vi "tracking2.vi"(4 "x 2":dbl=10.0, 6 "lane keep":bool, 7 "str_gain":dbl=0.9 format="%#_13g", 8 "Numeric 2":dbl=10.0 format="%#_13g", 9 "reset path":bool, 11 "xt":dbl) -> (3 "handle":dbl=-3.32529799262397)   [LabVIEW 2015]
uses:
  G_SEN.vi
  G_ALL.vi
  G_LCM.vi
panel:
  out "lanedist":dbl
  out "idxx":dbl[](array[numeric])
  out "idx":dbl
  in  "y 2":dbl=42.0
  out "XY Graph 2":cluster{"Y":dbl[], "Y":dbl[]}[](graph)=[{"Y"=array[11233 elements], "Y"=array[11233 elements]}, {"Y"=[-0.0, 0.0027755521495791413, 0.011103235155417224, 0.024986130588096955, 0.04442938073793812, 0.0694401981527264, 0.10002787904836907, 0.13620382065079895, 0.17798154254490584, 0.22537671212434418, 0.2784071742547809, 0.3370929852830926, 0.40145645154536425, 0.4715221725490224, 0.5473170890276435, 0.6288705360921867, 0.7162143017295008, 0.8093826909282242, 0.9084125957438758, 1.0133435716494645, 1.1242179205557647, 1.2410807809266515, 1.3639802254602955, 1.4929673668571652, 1.6280964722509026, 1.769425086939485, 1.9170141681219874, 2.0709282294217246, 2.2312354970611636, 2.3980080786478197, 2.5713221456362234], "Y"=[0.0, 0.5, 1.0, 1.5, 2.0, 2.5, 3.0, 3.5, 4.0, 4.5, 5.0, 5.5, 6.0, 6.5, 7.0, 7.5, 8.0, 8.5, 9.0, 9.5, 10.0, 10.5, 11.0, 11.5, 12.0, 12.5, 13.0, 13.5, 14.0, 14.5, 15.0]}, {"Y"=[-0.40885366553013214], "Y"=[0.1442103688222703]}, {"Y"=array[212 elements], "Y"=array[212 elements]}, {"Y"=[-0.925, -0.925, -0.925, -0.6775, -0.6775, -0.925, -0.925, -0.925, -0.925, -0.6775, -0.6775, -0.925, -0.925, -0.925, 0.9025, 0.9025, 0.9025, 0.6775, 0.6775, 0.9025, 0.9025, 0.9025, 0.9025, 0.6775, 0.6775, 0.9025, 0.9025, 0.9025, -0.925], "Y"=[-0.75, -0.224, 0.224, 0.224, -0.224, -0.224, 0.224, 2.415, 2.885, 2.885, 2.415, 2.415, 2.885, 3.5, 3.5, 2.885, 2.415, 2.415, 2.885, 2.885, 2.415, 0.224, -0.224, -0.224, 0.224, 0.224, -0.224, -0.75, -0.75]}, {"Y"=[0.0, 0.0, 0.0, 0.0, 0.0, 0.0, 0.0, 0.0, 0.0, 0.0], "Y"=[0.0, 0.5, 1.0, 1.5, 2.0, 2.5, 3.0, 3.5, 4.0, 4.5]}, {"Y"=[1.41796875, 1.3798326583616436, 1.3415997434556484, 1.3032752327956258, 1.2648643538951874, 1.226372334267944, 1.1878044014275073, 1.1491657828874886, 1.110461706161499, 1.07169739876315], "Y"=[0.0, 0.5, 1.0, 1.5, 2.0, 2.5, 3.0, 3.5, 4.0, 4.5]}, {"Y"=[-2.5234375, -2.5105986626297234, -2.4915998479127883, -2.466420726940036, -2.4350409708023073, -2.3974402505904435, -2.3535982373952864, -2.303494602307677, -2.247109016418457, -2.184421150818467], "Y"=[0.0, 0.5, 1.0, 1.5, 2.0, 2.5, 3.0, 3.5, 4.0, 4.5]}, {"Y"=[0.0, 0.0, 0.0, 0.0, 0.0, 0.0, 0.0, 0.0, 0.0, 0.0, 0.0, 0.0, 0.0, 0.0, 0.0, 0.0, 0.0, 0.0, 0.0, 0.0], "Y"=[0.0, 0.5, 1.0, 1.5, 2.0, 2.5, 3.0, 3.5, 4.0, 4.5, 5.0, 5.5, 6.0, 6.5, 7.0, 7.5, 8.0, 8.5, 9.0, 9.5]}]
  out "dist":dbl[](array[numeric])
  out "y origin":dbl[](array[numeric])
  out "x origin":dbl[](array[numeric])
  out "heading":dbl[](array[numeric])
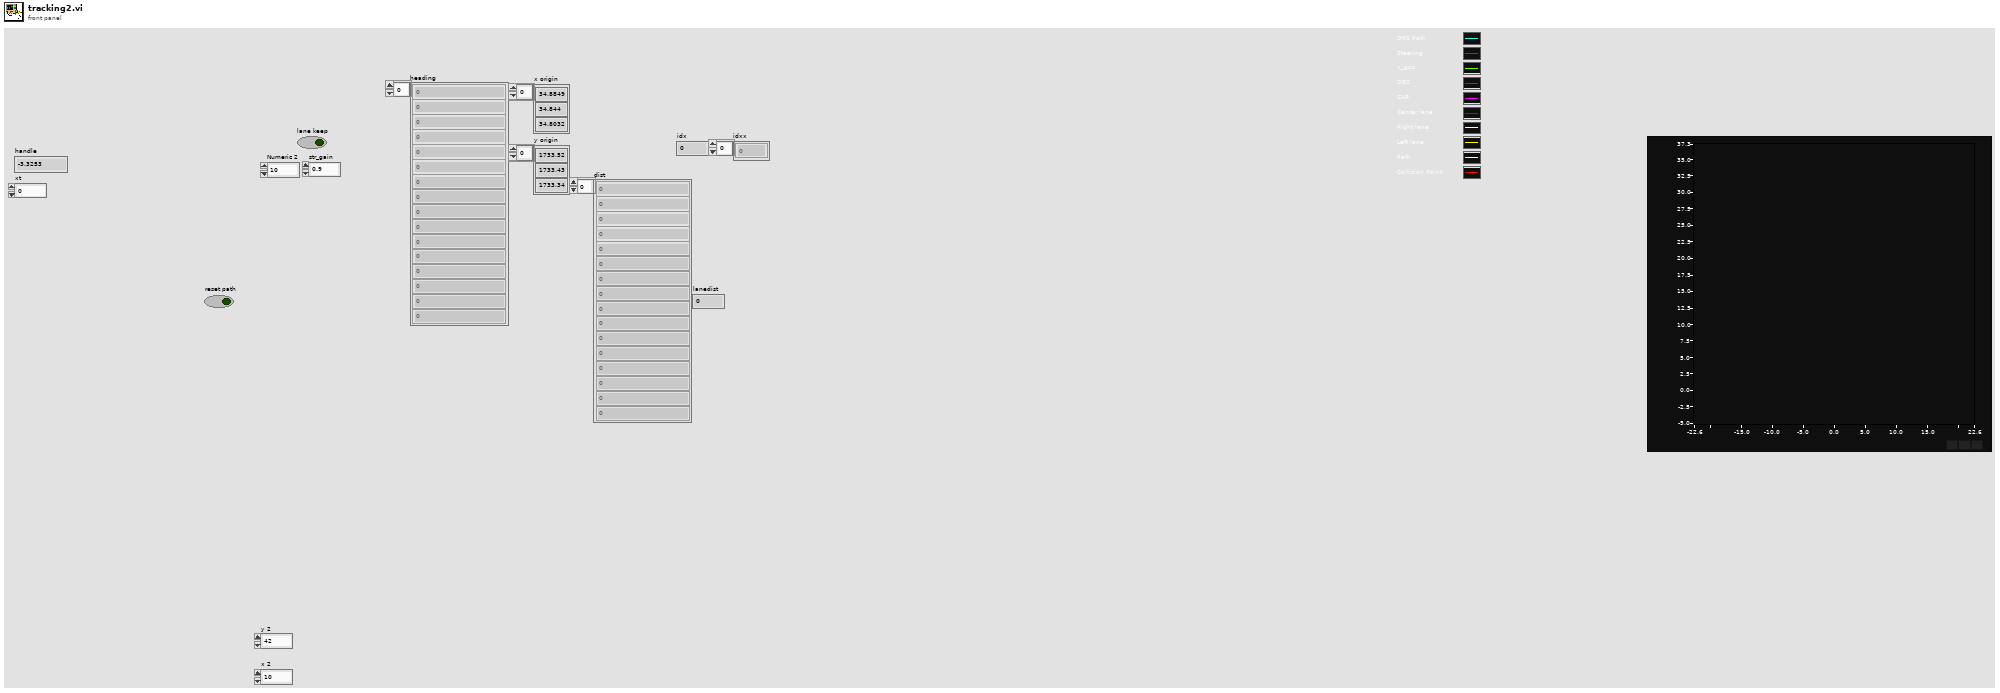
[diagram p1: front panel]
types:
  T1 = cluster{"Steer_input":dbl, "Steer_output":dbl, "VS_des":dbl, "VS_can":dbl, "heading":dbl, "auto":bool, "run":bool, "x":dbl, "y":dbl}
  T2 = cluster{"beep":bool, "duration (msec)":u32, "frequency (Hz)":u32}
  T3 = cluster{"C_Wheel base":dbl, "ratio_steer":dbl, "Overall width":dbl, "af":dbl, "turn radius":dbl, "eval":dbl, "ap":dbl, "an":dbl, "Vmax":dbl, "mu":dbl, "Vlast":dbl}
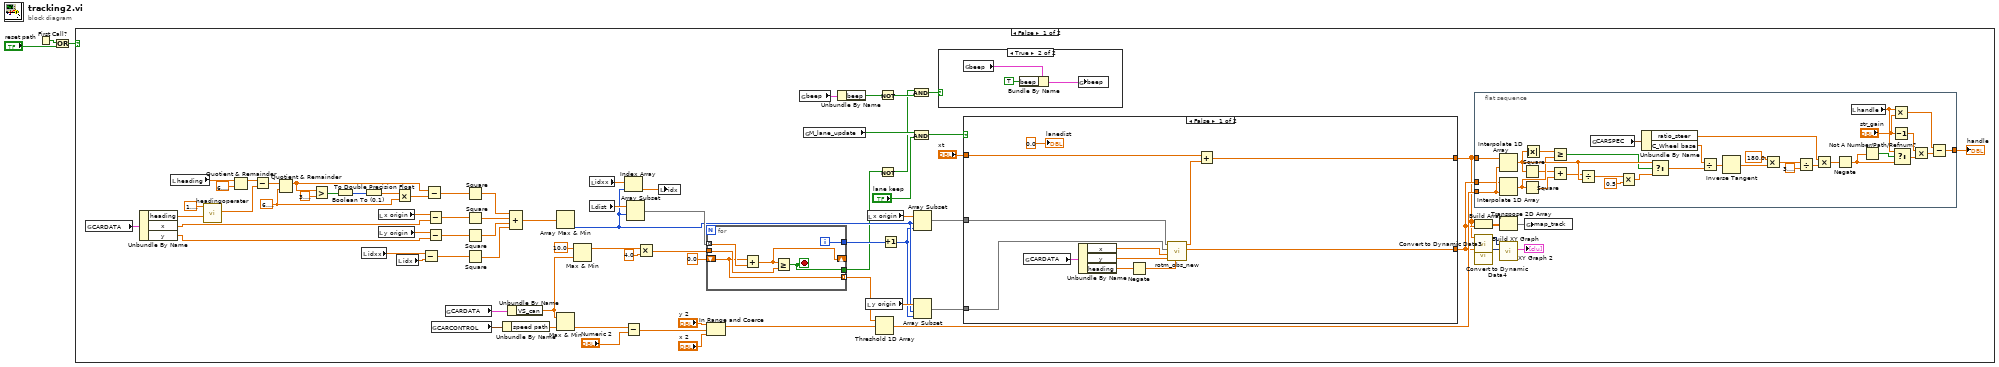
[diagram p0: block diagram]
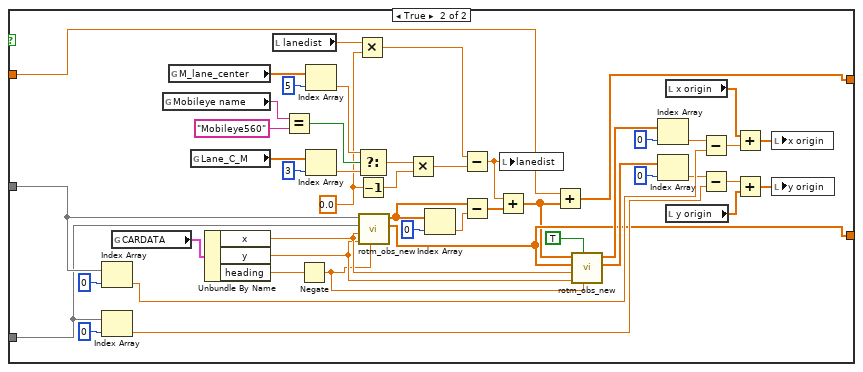
[diagram p3: hidden frame]
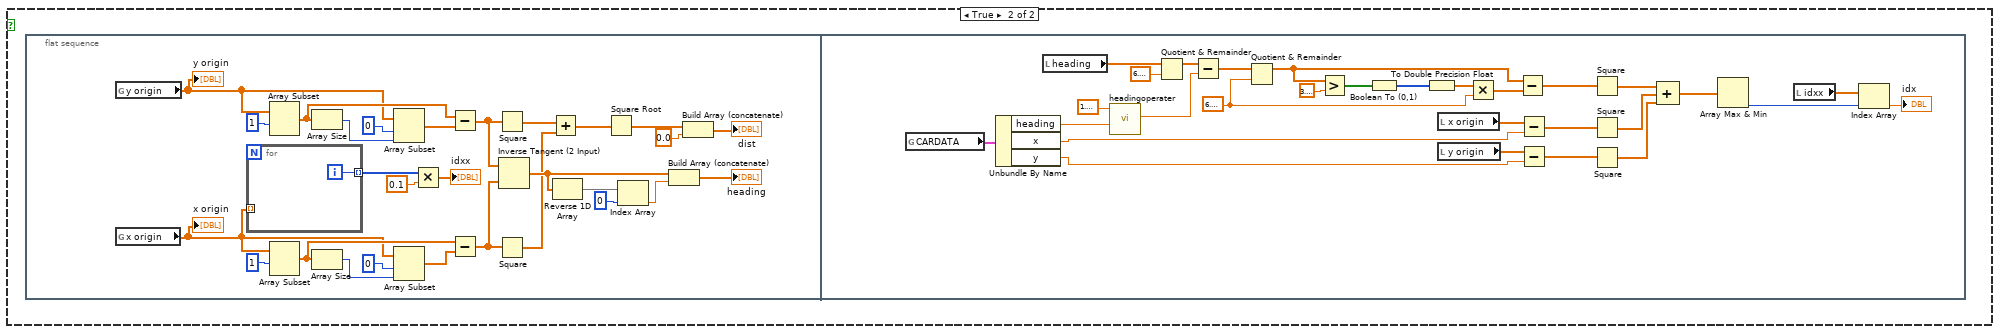
[diagram p4: hidden frame]
diagram:
  n1 = First Call?() -> (First Call?: T/F=w3:bool)
  n2 = Or(x=w3, y="reset path") -> (x .or. y?=w2:bool)
  n3 = case shown="False" w2 {
    frame False {
      w64 = 6.283185307179586
      n4 = global read "G_ALL.vi" "CARDATA"() -> (w11:T1)
      n5 = Unbundle By Name(w11) -> ("heading"=w58:dbl, "x"=w79:dbl, "y"=w77:dbl)
      n6 = local read "heading"() -> (w69:dbl[])
      n7 = call "headingoperater.vi"("h1"=w58, "h2"=1.5707963267948966) -> ("h2-h1"=w55:dbl)  [unwired: 8 in, 1 out]
      n8 = Quotient & Remainder(x=w69, y=6.283185307179586) -> (x-y*floor(x/y)=w70:dbl[])  [unwired: 1 out]
      n9 = Subtract(x=w70, y=w55) -> (x-y=w71:dbl[])
      n10 = Quotient & Remainder(x=w71, y=w64) -> (x-y*floor(x/y)=w72:dbl[])  [unwired: 1 out]
      n11 = Greater?(x=w72, y=3.141592653589793) -> (0:w68:bool[])
      n12 = Boolean To (0,1)(Boolean=w68) -> (0, 1=w67:i16[])
      n13 = local read "idxx"() -> (w25:dbl[])
      n14 = To Double Precision Float(number=w67) -> (double precision float=w65:dbl[])
      n15 = local read "x origin"() -> (w78:dbl[])
      n16 = local read "y origin"() -> (w76:dbl[])
      n17 = Multiply(x=w65, y=w64) -> (x*y=w66:dbl[])
      n18 = local read "idx"() -> (w26:dbl)
      n19 = Subtract(x=w25, y=w26) -> (x-y=w24:dbl[])
      n20 = Subtract(x=w72, y=w66) -> (x-y=w63:dbl[])
      n21 = Subtract(x=w78, y=w79) -> (x-y=w61:dbl[])
      n22 = Subtract(x=w76, y=w77) -> (x-y=w62:dbl[])
      n23 = global read "G_ALL.vi" "CARCONTROL"() -> (w5:cluster{"speed path":dbl, "speed limit":dbl})
      n24 = global read "G_ALL.vi" "CARDATA"() -> (w10:T1)
      n25 = Square(x=w63) -> (x^2=w60:dbl[])
      n26 = Square(x=w61) -> (x^2=w57:dbl[])
      n27 = Square(x=w62) -> (x^2=w56:dbl[])
      n28 = Square(x=w24) -> (x^2=w23:dbl[])
      n29 = Unbundle By Name(w5) -> ("speed path"=w4:dbl)
      n30 = Unbundle By Name(w10) -> ("VS_can"=w9:dbl)
      n31 = Compound Arithmetic op=ADD(w60, w57, w56, w23) -> (w59:dbl[])
      n32 = Array Max & Min(array=w59) -> (min index (indices)=w21:i32)  [unwired: 3 out]
      n33 = Max & Min(x=w9, y=w4) -> (min(x,y)=w29:dbl)  [unwired: 1 out]
      n34 = Max & Min(x=10.0, y=w9) -> (max(x,y)=w52:dbl)  [unwired: 1 out]
      n35 = local read "idxx"() -> (w22:dbl[])
      n36 = local read "dist"() -> (w54:dbl[])
      n37 = Index Array(array=w22, index=w21) -> (element=w20:dbl)
      n38 = Subtract(x=w29, y="Numeric 2") -> (x-y=w28:dbl)
      n39 = Array Subset(array=w54, index=w21) -> (w50:dbl[])  [unwired: 1 in]
      n40 = Multiply(x=w52, y=4.0) -> (x*y=w49:dbl)
      n41 = local write "idx"(w20) -> ()
      n42 = for {
        tunnel: w50 -> [w181] mode=indexing
        tunnel: w49 -> [w179]
        shift-right: [w180] -> _
        shift-left: 0.0 -> [w177]
        tunnel: [w178] -> w47
        tunnel: [w177] -> w31 mode=indexing
        tunnel: [w176] -> w13
        i -> [w178]
        stop <- w176 stop-if-true
        n43 = Add(x=w177, y=w181) -> (x+y=w180:dbl)
        n44 = Greater Or Equal?(x=w180, y=w179) -> (x >= y?=w176:bool)
      }
      n45 = In Range and Coerce(upper limit="y 2", x=w28, lower limit="x 2") -> (coerced(x)=w36:dbl)  [unwired: 1 out]
      n46 = global read "G_ALL.vi" "beep"() -> (w7:T2)
      n47 = global read "G_SEN.vi" "M_lane_update"() -> (w42:bool)
      n48 = Unbundle By Name(w7) -> ("beep"=w6:bool)
      n49 = local read "y origin"() -> (w43:dbl[])
      n50 = local read "x origin"() -> (w44:dbl[])
      n51 = Threshold 1D Array(2:w36, 3:w31) -> (0:w37:dbl)  [unwired: 1 in]
      n52 = Not(x=w6) -> (.not. x?=w17:bool)
      n53 = Not(x=w13) -> (.not. x?=w12:bool)
      n54 = Increment(x=w47) -> (x+1=w14:i32)
      n55 = And(x=w12, y=w17) -> (x .and. y?=w16:bool)
      n56 = And(x=w42, y="lane keep") -> (x .and. y?=w41:bool)
      n57 = Array Subset(array=w44, index=w21, length=w14) -> (w46:dbl[])
      n58 = Array Subset(array=w43, index=w21, length=w14) -> (w15:dbl[])
      n59 = case shown="True" w16 {
        frame False {
        }
        frame True {
          n60 = global read "G_ALL.vi" "beep"() -> (w82:T2)
          n61 = Bundle By Name(cluster=w82, "beep"=TRUE) -> (w81:T2)
          n62 = global write "G_ALL.vi" "beep"(w81) -> ()
        }
      }
      n63 = case shown="False" w41 {
        tunnel: w46 -> [w123 w154]
        tunnel: w15 -> [w122 w152]
        tunnel: [w120 w137] -> w32
        tunnel: [w121 w139] -> w33
        tunnel: "xt" -> [w118 w136]
        frame False {
          n64 = global read "G_ALL.vi" "CARDATA"() -> (w116:T1)
          n65 = Unbundle By Name(w116) -> ("x"=w126:dbl, "y"=w125:dbl, "heading"=w127:dbl)
          n66 = Negate(x=w127) -> (-x=w124:dbl)
          n67 = call "rotm_obs_new.vi"("angle[rad]"=w124, "y0"=w125, "x0"=w126, "y"=w122, "x"=w123) -> ("rot*(y-y0) 2"=w121:dbl[], "rot*(x-x0)"=w119:dbl[])  [unwired: 3 in, 2 out]
          n68 = Add(x=w118, y=w119) -> (x+y=w120:dbl[])
          "lanedist" <- 0.0
        }
        frame True {
          w134 = 0.0 ("x")
          n69 = Index Array(array=w154, index=0) -> (element=w150:dbl)
          n70 = Index Array(array=w152, index=0) -> (element=w146:dbl)
          n71 = global read "G_ALL.vi" "CARDATA"() -> (w128:T1)
          n72 = global read "G_LCM.vi" "Mobileye name"() -> (w167:string)
          n73 = global read "G_SEN.vi" "M_lane_center"() -> (w162:dbl[])
          n74 = global read "G_SEN.vi" "Lane_C_M"() -> (w169:dbl[])
          n75 = Unbundle By Name(w128) -> ("x"=w160:dbl, "y"=w159:dbl, "heading"=w175:dbl)
          n76 = local read "lanedist"() -> (w135:dbl)
          n77 = Equal?(x=w167, y="Mobileye560") -> (x = y?=w165:bool)
          n78 = Negate(x=w175) -> (-x=w158:dbl)
          n79 = Index Array(array=w162, index=5) -> (element=w161:dbl)
          n80 = Index Array(array=w169, index=3) -> (element=w164:dbl)
          n81 = Multiply(x=w135, y=w134) -> (x*y=w131:dbl)
          n82 = Select(t=w161, s=w165, f=w164) -> (s? t:f=w133:dbl)
          n83 = Decrement(x=w134) -> (x-1=w132:dbl)
          n84 = call "rotm_obs_new.vi"("angle[rad]"=w158, "y0"=w159, "x0"=w160, "y"=w152, "x"=w154) -> ("rot*(y-y0) 2"=w139:dbl[], "rot*(x-x0)"=w172:dbl[])  [unwired: 3 in, 2 out]
          n85 = Multiply(x=w133, y=w132) -> (x*y=w130:dbl)
          n86 = Index Array(array=w172, index=0) -> (element=w173:dbl)
          n87 = Subtract(x=w131, y=w130) -> (x-y=w129:dbl)
          n88 = Subtract(x=w172, y=w173) -> (x-y=w171:dbl[])
          n89 = Add(x=w129, y=w171) -> (x+y=w138:dbl[])
          n90 = local write "lanedist"(w129) -> ()
          n91 = Add(x=w136, y=w138) -> (x+y=w137:dbl[])
          n92 = call "rotm_obs_new.vi"("angle[rad]"=w158, "reverse"=TRUE, "y0"=w159, "x0"=w160, "y"=w139, "x"=w138) -> ("rot*(y-y0) 2"=w148:dbl[], "rot*(x-x0)"=w157:dbl[])  [unwired: 2 in, 2 out]
          n93 = Index Array(array=w157, index=0) -> (element=w151:dbl)
          n94 = Index Array(array=w148, index=0) -> (element=w147:dbl)
          n95 = local read "x origin"() -> (w144:dbl[])
          n96 = local read "y origin"() -> (w142:dbl[])
          n97 = Subtract(x=w151, y=w150) -> (x-y=w145:dbl)
          n98 = Subtract(x=w147, y=w146) -> (x-y=w143:dbl)
          n99 = Add(x=w144, y=w145) -> (x+y=w141:dbl[])
          n100 = Add(x=w143, y=w142) -> (x+y=w140:dbl[])
          n101 = local write "x origin"(w141) -> ()
          n102 = local write "y origin"(w140) -> ()
        }
      }
      n103 = flat-sequence {
        tunnel: w37 -> [w113]
        tunnel: w33 -> [w112]
        tunnel: w32 -> [w93]
        tunnel: [w86] -> w30
        frame #0 {
          n104 = Interpolate 1D Array(1:w113, 2:w93) -> (0:w115:dbl)
          n105 = Interpolate 1D Array(1:w113, 2:w112) -> (0:w114:dbl)
          n106 = Square(x=w115) -> (x^2=w98:dbl)
          n107 = Square(x=w114) -> (x^2=w99:dbl)
          n108 = Absolute Value(x=w115) -> (abs(x)=w97:dbl)
          n109 = Greater Or Equal?(x=w97, y=w114) -> (x >= y?=w96:bool)
          n110 = Add(x=w98, y=w99) -> (x+y=w100:dbl)
          n111 = Divide(x=w100, y=w115) -> (x/y=w101:dbl)
          n112 = global read "G_ALL.vi" "CARSPEC"() -> (w85:T3)
          n113 = Multiply(x=w101, y=0.5) -> (x*y=w103:dbl)
          n114 = Unbundle By Name(w85) -> ("ratio_steer"=w84:dbl, "C_Wheel base"=w83:dbl)
          n115 = Select(t=w115, s=w96, f=w103) -> (s? t:f=w104:dbl)
          n116 = Divide(x=w83, y=w104) -> (x/y=w105:dbl)
          n117 = Inverse Tangent(1:w105) -> (0:w107:dbl)
          n118 = Multiply(x=180.0 ("y"), y=w107) -> (x*y=w108:dbl)
          n119 = Divide(x=w108, y=3.141592653589793) -> (x/y=w110:dbl)
          n120 = Multiply(x=w84, y=w110) -> (x*y=w111:dbl)
          n121 = Negate(x=w111) -> (-x=w94:dbl)
          n122 = local read "handle"() -> (w92:dbl)
          n123 = Not A Number/Path/Refnum?(number/path/refnum=w94) -> (NaN/Path/Refnum?=w95:bool)
          n124 = Multiply(x=w92, y="str_gain") -> (x*y=w88:dbl)
          n125 = Decrement(x="str_gain") -> (x-1=w90:dbl)
          n126 = Select(t=w92, s=w95, f=w94) -> (s? t:f=w89:dbl)
          n127 = Multiply(x=w90, y=w89) -> (x*y=w87:dbl)
          n128 = Subtract(x=w88, y=w87) -> (x-y=w86:dbl)
        }
      }
      n129 = Build Array(w32, w33) -> (w38:dbl[][])
      n130 = call "Convert to Dynamic Data3"("Array"=w32) -> ("Dynamic Data Type"=w40:dynamicdata)  [unwired: 3 in]
      n131 = call "Convert to Dynamic Data4"("Array"=w33) -> ("Dynamic Data Type"=w39:dynamicdata)  [unwired: 3 in]
      n132 = Transpose 2D Array(2D array=w38) -> (transposed array=w8:dbl[][])
      n133 = call "Build XY Graph"("Y Input"=w39, "X Input"=w40) -> ("XY Graph"=→"XY Graph 2":cluster{"X":dbl[], "Y":dbl[]}[])  [unwired: 8 in, 1 out]
      n134 = global write "G_ALL.vi" "map_track"(w8) -> ()
      "handle" <- w30
    }
    frame True {
      n135 = flat-sequence {
        frame #0 {
          n136 = global read "G_ALL.vi" "y origin"() -> (w182:dbl[])
          "y origin" <- w182
          n137 = global read "G_ALL.vi" "x origin"() -> (w183:dbl[])
          "x origin" <- w183
          n138 = for {
            tunnel: w183 -> [_] mode=indexing
            tunnel: [w210] -> w186 mode=indexing
            i -> [w210]
          }
          n139 = Array Subset(array=w182, index=1) -> (w204:dbl[])  [unwired: 1 in]
          n140 = Array Subset(array=w183, index=1) -> (w205:dbl[])  [unwired: 1 in]
          n141 = Array Size(array=w204) -> (size(s)=w201:i32)
          n142 = Array Size(array=w205) -> (size(s)=w208:i32)
          n143 = Array Subset(array=w182, index=0, length=w201) -> (w203:dbl[])
          n144 = Array Subset(array=w183, index=0, length=w208) -> (w206:dbl[])
          n145 = Multiply(x=w186, y=0.1) -> (x*y=→"idxx":dbl[])
          n146 = Subtract(x=w204, y=w203) -> (x-y=w194:dbl[])
          n147 = Subtract(x=w205, y=w206) -> (x-y=w193:dbl[])
          n148 = Square(x=w194) -> (x^2=w192:dbl[])
          n149 = Square(x=w193) -> (x^2=w191:dbl[])
          n150 = Inverse Tangent (2 Input)(1:w193, 2:w194) -> (0:w195:dbl[])
          n151 = Add(x=w192, y=w191) -> (x+y=w190:dbl[])
          n152 = Reverse 1D Array(array=w195) -> (reversed array=w199:dbl[])
          n153 = Square Root(x=w190) -> (sqrt(x)=w189:dbl[])
          n154 = Index Array(array=w199, index=0) -> (element=w197:dbl)
          n155 = Build Array (concatenate)(w195, w197) -> (→"heading":dbl[])
          n156 = Build Array (concatenate)(w189, 0.0) -> (→"dist":dbl[])
        }
        frame #1 {
          w224 = 6.283185307179586
          n157 = global read "G_ALL.vi" "CARDATA"() -> (w211:T1)
          n158 = Unbundle By Name(w211) -> ("heading"=w218:dbl, "x"=w239:dbl, "y"=w237:dbl)
          n159 = local read "heading"() -> (w229:dbl[])
          n160 = call "headingoperater.vi"("h1"=w218, "h2"=1.5707963267948966) -> ("h2-h1"=w215:dbl)  [unwired: 8 in, 1 out]
          n161 = Quotient & Remainder(x=w229, y=6.283185307179586) -> (x-y*floor(x/y)=w230:dbl[])  [unwired: 1 out]
          n162 = Subtract(x=w230, y=w215) -> (x-y=w231:dbl[])
          n163 = Quotient & Remainder(x=w231, y=w224) -> (x-y*floor(x/y)=w232:dbl[])  [unwired: 1 out]
          n164 = Greater?(x=w232, y=3.141592653589793) -> (0:w228:bool[])
          n165 = Boolean To (0,1)(Boolean=w228) -> (0, 1=w227:i16[])
          n166 = To Double Precision Float(number=w227) -> (double precision float=w225:dbl[])
          n167 = local read "x origin"() -> (w238:dbl[])
          n168 = local read "y origin"() -> (w236:dbl[])
          n169 = Multiply(x=w225, y=w224) -> (x*y=w226:dbl[])
          n170 = Subtract(x=w232, y=w226) -> (x-y=w223:dbl[])
          n171 = Subtract(x=w238, y=w239) -> (x-y=w221:dbl[])
          n172 = Subtract(x=w236, y=w237) -> (x-y=w222:dbl[])
          n173 = Square(x=w223) -> (x^2=w220:dbl[])
          n174 = Square(x=w221) -> (x^2=w217:dbl[])
          n175 = Square(x=w222) -> (x^2=w216:dbl[])
          n176 = Compound Arithmetic op=ADD(w220, w217, w216) -> (w219:dbl[])
          n177 = Array Max & Min(array=w219) -> (min index (indices)=w213:i32)  [unwired: 3 out]
          n178 = local read "idxx"() -> (w214:dbl[])
          n179 = Index Array(array=w214, index=w213) -> (element=→"idx":dbl)
        }
      }
    }
  }
